vi "Notes_moyennes.vi"() -> ()   [LabVIEW 2018]
panel:
  out "Tableau":dbl[](array[numeric])
  in  "Note 6":i8=3 min=1 max=6
  in  "Note 5":i8=3 min=3 max=6
  in  "Note 4":i8=3 min=3 max=6
  in  "Note 3":i8=3 min=3 max=6
  in  "Note 2":i8=3 min=3 max=6
  in  "Note 1":i8=3 min=3 max=6
  out "Moyenne visée":dbl format="%^#_6g"
  out "Moyenne actuelle":dbl
  in  "stop":bool
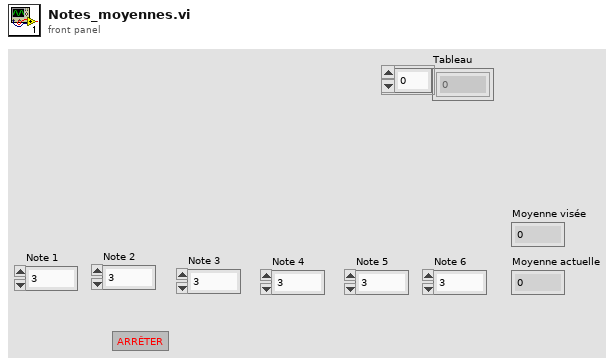
[diagram p1: front panel]
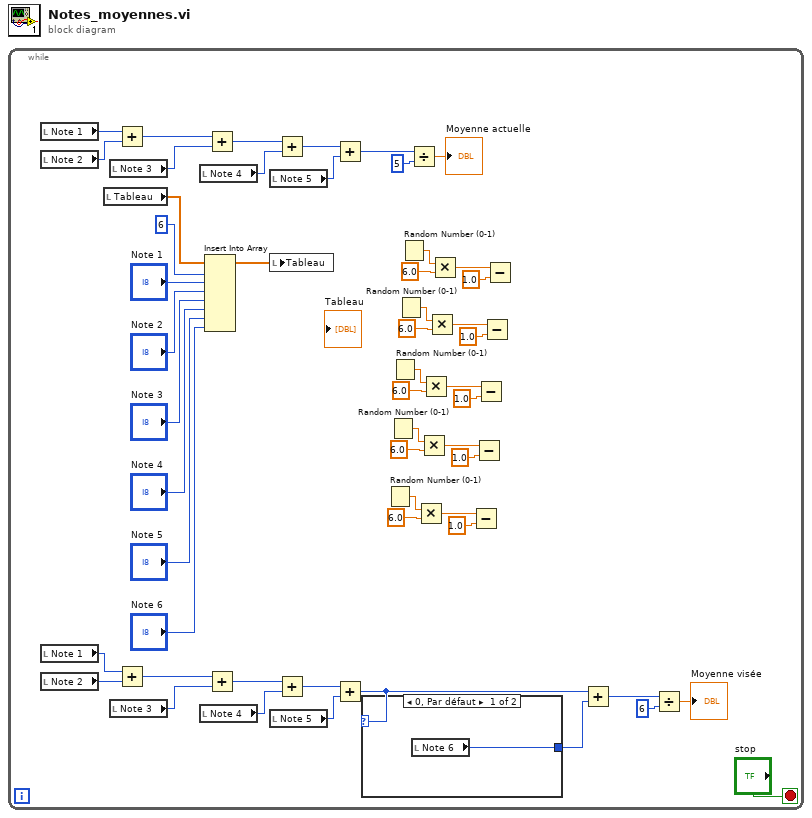
[diagram p0: block diagram]
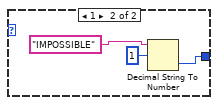
[diagram p2: hidden frame]
diagram:
  n1 = while {
    stop <- "stop" stop-if-true
    n2 = local read "Note 1"() -> (w29:i8)
    n3 = local read "Note 2"() -> (w30:i8)
    n4 = local read "Note 1"() -> (w47:i8)
    n5 = local read "Note 2"() -> (w48:i8)
    n6 = local read "Tableau"() -> (w19:dbl[])
    n7 = local read "Note 3"() -> (w31:i8)
    n8 = local read "Note 3"() -> (w49:i8)
    n9 = Add(x=w29, y=w30) -> (x+y=w26:i8)
    n10 = Add(x=w47, y=w48) -> (x+y=w42:i8)
    n11 = local read "Note 4"() -> (w32:i8)
    n12 = local read "Note 4"() -> (w50:i8)
    n13 = Insert Into Array(array=w19, index=6 ("indice"), new element #1="Note 1", new element #2="Note 2", new element #3="Note 3", new element #4="Note 4", new element #5="Note 5", new element #6="Note 6") -> (w20:dbl[])
    n14 = Add(x=w26, y=w31) -> (x+y=w27:i8)
    n15 = Add(x=w42, y=w49) -> (x+y=w43:i8)
    n16 = local read "Note 5"() -> (w33:i8)
    n17 = local write "Tableau"(w20) -> ()
    n18 = local read "Note 5"() -> (w51:i8)
    n19 = Add(x=w27, y=w32) -> (x+y=w28:i8)
    n20 = Add(x=w43, y=w50) -> (x+y=w44:i8)
    n21 = Add(x=w28, y=w33) -> (x+y=w23:i8)
    n22 = Add(x=w44, y=w51) -> (x+y=w40:i8)
    n23 = case shown="0, Par défaut" w40 {
      tunnel: [w55 w56] -> w1
      frame 0, Default {
        n24 = local read "Note 6"() -> (w55:i8)
      }
      frame 1 {
        n25 = Decimal String To Number(string="IMPOSSIBLE", offset=1) -> (number=w56:i32)  [unwired: 1 in, 1 out]
      }
    }
    n26 = Random Number (0-1)() -> (number: 0 to 1=w5:dbl)
    n27 = Random Number (0-1)() -> (number: 0 to 1=w9:dbl)
    n28 = Random Number (0-1)() -> (number: 0 to 1=w13:dbl)
    n29 = Random Number (0-1)() -> (number: 0 to 1=w17:dbl)
    n30 = Random Number (0-1)() -> (number: 0 to 1=w53:dbl)
    n31 = Divide(x=w23, y=i8 5) -> (x/y=→"Moyenne actuelle":dbl)
    n32 = Multiply(x=w5, y=6.0) -> (x*y=w2:dbl)
    n33 = Multiply(x=w9, y=6.0) -> (x*y=w6:dbl)
    n34 = Multiply(x=w13, y=6.0) -> (x*y=w10:dbl)
    n35 = Multiply(x=w17, y=6.0) -> (x*y=w14:dbl)
    n36 = Multiply(x=w53, y=6.0) -> (x*y=w21:dbl)
    n37 = Subtract(x=w2, y=1.0) -> ()  [unwired: 1 out]
    n38 = Subtract(x=w6, y=1.0) -> ()  [unwired: 1 out]
    n39 = Subtract(x=w10, y=1.0) -> ()  [unwired: 1 out]
    n40 = Subtract(x=w14, y=1.0) -> ()  [unwired: 1 out]
    n41 = Subtract(x=w21, y=1.0) -> ()  [unwired: 1 out]
    n42 = Add(x=w40, y=w1) -> (x+y=w45:i32)
    n43 = Divide(x=w45, y=i8 6) -> (x/y=→"Moyenne visée":dbl)
  }
